vi "Enable Micro Wave Preselector Bypass.vi"(0 "VISA resource name":refnum<visa-resource-name>, 5 "Enable Preselector Bypass (0:Disable)":bool, 11 "error in (no error)":errorcluster) -> (4 "VISA resource name out":refnum<visa-resource-name>, 15 "error out":errorcluster)   [LabVIEW 2020, in "Anritsu Signal Analyzer Series.lvlib"]
doc: "Configures the Micro Wave Preselector Bypass settings of the spectrum analyzer."
uses:
  Anritsu Signal Analyzer Series.lvlib
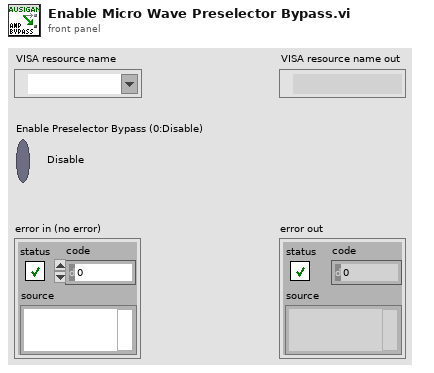
[diagram p1: front panel]
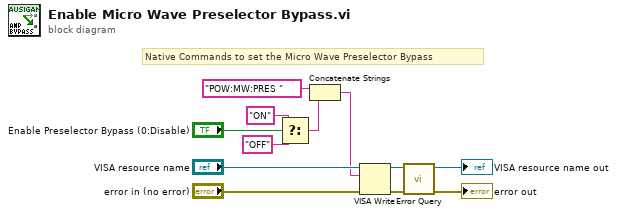
[diagram p0: block diagram]
diagram:
  # "Native Commands to set the Micro Wave Preselector Bypass"
  n1 = Select(t="ON" ("複数行文字列"), s="Enable Preselector Bypass (0:Disable)", f="OFF" ("複数行文字列")) -> (s? t:f=w1:string)
  n2 = Concatenate Strings("POW:MW:PRES " ("_CommandSet"), w1) -> (w4:string)
  n3 = VISA Write(VISA resource name="VISA resource name", write buffer=w4, error in (no error)="error in (no error)") -> (VISA resource name out=w7:refnum<visa-resource-name>, error out=w8:errorcluster)  [unwired: 1 out]
  n4 = call "Error Query.vi"("error in (no error)"=w8, "VISA resource name"=w7) -> ("error out"=→"error out":errorcluster, "VISA resource name out"=→"VISA resource name out":refnum<visa-resource-name>)  [unwired: 6 in, 2 out]
